vi "CallbackY.vi"(11 "IRQ Number":u8) -> ()   [LabVIEW 2017]
uses:
  <vilib>/myRIO/Instrument Drivers/Onboard IO/DIO/typedefs/DIO Reference.ctl
  <vilib>/myRIO/Common/Instrument Driver Framework/Utilities/typedefs/myRIO Generic Hardware Reference.ctl
  <vilib>/myRIO/Common/Instrument Driver Framework/Utilities/typedefs/Hardware Version Enum.ctl
  <vilib>/myRIO/Common/Instrument Driver Framework/Utilities/typedefs/myRIO v1.0 Reference.ctl
  <vilib>/myRIO/Common/Instrument Driver Framework/Utilities/typedefs/Generic FPGA Reference.ctl
  <vilib>/myRIO/Common/Instrument Driver Framework/myRIO v1.0/DIO/typedefs/DIO Channels List.ctl
  <vilib>/myRIO/Common/Instrument Driver Framework/myRIO v1.0/DIO/typedefs/DIO Channels Enum.ctl
  <vilib>/userdefined/High Color/nirio_resource_hc.ctl
  <vilib>/myRIO/Instrument Drivers/Onboard IO/DIO/vis/Write.vi
  <vilib>/myRIO/Common/Instrument Driver Framework/myRIO v1.0/DIO/vis/myRIO v1.1 Open DIO.vi
  <vilib>/myRIO/Common/Instrument Driver Framework/Utilities/vis/Is FPGA Ref Available.vi
  <vilib>/myRIO/Common/Instrument Driver Framework/Utilities/vis/Validate Channels.vi
  <vilib>/myRIO/Common/Instrument Driver Framework/myRIO v1.0/DIO/vis/myRIO v1.0 Reserve DIO.vi
  <vilib>/myRIO/Common/Instrument Driver Framework/myRIO v1.0/Resource Manager/vis/myRIO v1.0 Reserve Channel List.vi
  <vilib>/myRIO/Common/Instrument Driver Framework/myRIO v1.0/DIO/vis/myRIO v1.0 Build MUX Configuration DIO.vi
  <vilib>/myRIO/Common/Instrument Driver Framework/myRIO v1.0/Resource Manager/vis/myRIO v1.0 Reserve Channel.vi
  <vilib>/myRIO/Common/Instrument Driver Framework/myRIO v1.0/Resource Manager/vis/myRIO v1.0 Unreserve Channel.vi
  <vilib>/myRIO/Common/Instrument Driver Framework/myRIO v1.0/Resource Manager/vis/myRIO v1.0 Create Configuration List.vi
  <vilib>/myRIO/Common/Instrument Driver Framework/myRIO v1.0/Resource Manager/vis/myRIO v1.0 Build Mutex Name.vi
  <vilib>/myRIO/Common/Instrument Driver Framework/myRIO v1.0/DIO/vis/myRIO v1.0 Write DIO.vi
  <vilib>/Utility/error.llb/Error Cluster From Error Code.vi
  <vilib>/myRIO/Common/Instrument Driver Framework/myRIO v1.0/myRIO v1.0 Close.vi
  <vilib>/myRIO/Common/Instrument Driver Framework/myRIO v1.0/Resource Manager/vis/myRIO v1.0 Configure IO.vi
  <vilib>/myRIO/Common/Instrument Driver Framework/Utilities/vis/IO Manager.vi
  <vilib>/myRIO/Common/Instrument Driver Framework/Utilities/vis/Configuration Manager.vi
  <vilib>/myRIO/Common/Instrument Driver Framework/myRIO v1.0/myRIO v1.1 Open.vi
  <vilib>/Utility/VariantDataType/GetNumericInfo.vi
  Globales.vi
  <vilib>/myRIO/Instrument Drivers/Onboard IO/DIO/vis/myRIO DIO Open.xnode
  <vilib>/myRIO/Express VI/Onboard IO/DO/DO Express VI.xnode
  <vilib>/myRIO/Instrument Drivers/Onboard IO/DIO/DIO.lvlib
panel:
  out "Stop?":bool
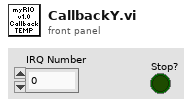
[diagram p1: front panel]
types:
  T1 = typedef "DIO.lvlib/DIO Reference.ctl" = cluster{"myRIO Reference":T2, "DIO Channels List":T6}
  T2 = typedef "myRIO Generic Hardware Reference.ctl" = cluster{"myRIO Model":T3, "myRIO Hardware Reference":T4}
  T3 = typedef "Hardware Version Enum.ctl" = enum16{"Unknown", "myRIO-1900", "myRIO-1950", "roboRIO", "NI ELVIS RIO CM"}
  T4 = typedef "myRIO v1.0 Reference.ctl" = cluster{"Generic FPGA Reference":T5, "Allow multiple opens":bool}
  T5 = typedef "Generic FPGA Reference.ctl" = refnum<k20>
  T6 = typedef "DIO Channels List.ctl" = T7[]
  T7 = typedef "DIO Channels Enum.ctl" = enum16{"Not Connected", "C/DIO0", "C/DIO1", "C/DIO2", "C/DIO3", "C/DIO4", "C/DIO5", "C/DIO6", "C/DIO7", "A/DIO0", "A/DIO1", "A/DIO2", "A/DIO3", "A/DIO4", "A/DIO5", "A/DIO6", "A/DIO7", "A/DIO8", "A/DIO9", "A/DIO10", "A/DIO11", "A/DIO12", "A/DIO13", "A/DIO14", "A/DIO15", "B/DIO0", "B/DIO1", "B/DIO2", "B/DIO3", "B/DIO4", "B/DIO5", "B/DIO6", "B/DIO7", "B/DIO8", "B/DIO9", "B/DIO10", "B/DIO11", "B/DIO12", "B/DIO13", "B/DIO14", "B/DIO15", "LED0", "LED1", "LED2", "LED3", "Button0", "DIO/DIO0", "DIO/DIO1", "DIO/DIO2", "DIO/DIO3", "DIO/DIO4", "DIO/DIO5", "DIO/DIO6", "DIO/DIO7", "DIO/DIO8", "DIO/DIO9", "SPI/CS0", "SPI/CS1", "SPI/CS2", "SPI/CS3", "LED RADIO (Green)", "LED RADIO (Red)", "LED COMM (Green)", "LED COMM (Red)", "LED MODE (Green)", "LED MODE (Red)"}
  T8 = typedef "nirio_resource_hc.ctl" = tag
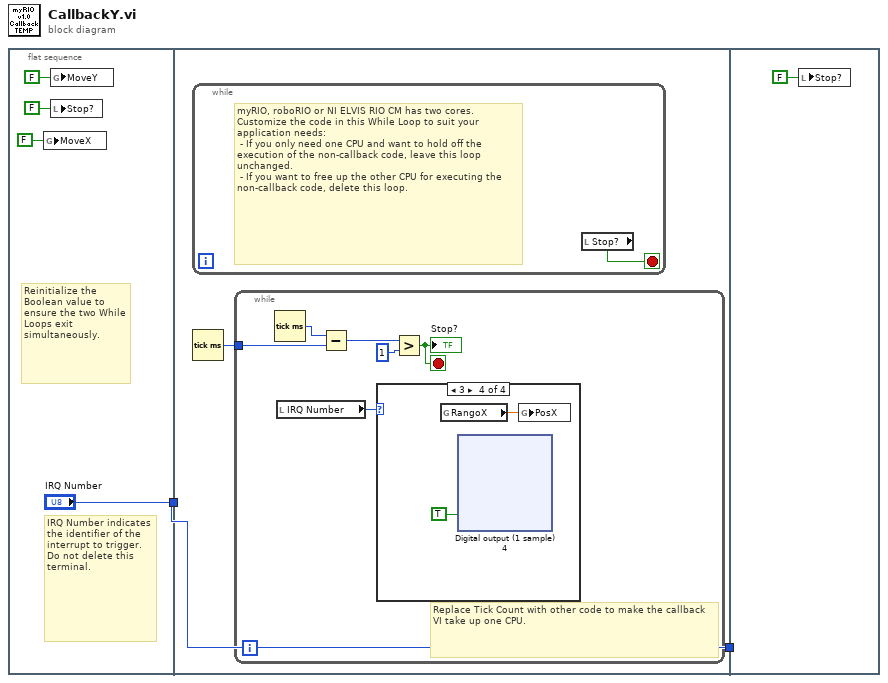
[diagram p0: block diagram]
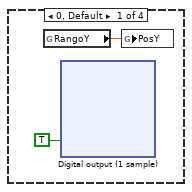
[diagram p2: hidden frame]
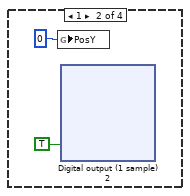
[diagram p3: hidden frame]
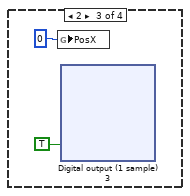
[diagram p4: hidden frame]
diagram:
  n1 = flat-sequence {
    tunnel: ["IRQ Number"] -> w2
    tunnel: [w8] -> w1
    tunnel: w2 -> [w8]
    tunnel: w1 -> [_]
    frame #0 {
      # "Reinitialize the Boolean value to ensure the two While Loops exit simultaneously."
      # "IRQ Number indicates the identifier of the interrupt to trigger. Do not delete this terminal."
      n2 = global write "Globales.vi" "MoveX"(FALSE) -> ()
      n3 = global write "Globales.vi" "MoveY"(FALSE) -> ()
      n4 = local write "Stop?"(FALSE ("Stop?")) -> ()
    }
    frame #1 {
      n5 = while {
        stop <- w9 stop-if-true
        # "myRIO, roboRIO or NI ELVIS RIO CM has two cores. Customize the code in this While Loop to suit your application needs:\n - If you only need one CPU and want to hold off the execution of the non-callback code, leave this loop unchanged.\n - If you want to free up the other CPU for executing the non-callback code, delete this loop."
        n6 = local read "Stop?"() -> (w9:bool)
      }
      n7 = Tick Count (ms)() -> (millisecond timer value=w7:u32)
      n8 = while {
        tunnel: w7 -> [w12]
        stop <- w11 stop-if-true
        # "Replace Tick Count with other code to make the callback VI take up one CPU."
        n9 = Tick Count (ms)() -> (millisecond timer value=w13:u32)
        n10 = local read "IRQ Number"() -> (w10:u8)
        n11 = Subtract(x=w13, y=w12) -> (x-y=w14:u32)
        n12 = case shown="3" w10 {
          frame 0, Default {
            n13 = global read "Globales.vi" "RangoY"() -> (w17:dbl)
            n14 = xnode "Digital output (1 sample)"("ON/OFF Y (A/DIO7 (Pin 25))"=TRUE) -> ()  [unwired: 1 in, 1 out]
            n15 = global write "Globales.vi" "PosY"(w17) -> ()
          }
          frame 1 {
            n16 = global write "Globales.vi" "PosY"(0) -> ()
            n17 = xnode "Digital output (1 sample) 2"("ON/OFF Y (A/DIO7 (Pin 25))"=TRUE) -> ()  [unwired: 1 in, 1 out]
          }
          frame 2 {
            n18 = global write "Globales.vi" "PosX"(0) -> ()
            n19 = xnode "Digital output (1 sample) 3"("ON/OFF Y (A/DIO4 (Pin 19))"=TRUE) -> ()  [unwired: 1 in, 1 out]
          }
          frame 3 {
            n20 = global read "Globales.vi" "RangoX"() -> (w128:dbl)
            n21 = xnode "Digital output (1 sample) 4"("ON/OFF X (A/DIO4 (Pin 19))"=TRUE) -> ()  [unwired: 1 in, 1 out]
            n22 = global write "Globales.vi" "PosX"(w128) -> ()
          }
        }
        n23 = Greater?(x=w14, y=u32 1) -> (0:w11:bool)
        "Stop?" <- w11
      }
    }
    frame #2 {
      n24 = local write "Stop?"(FALSE) -> ()
    }
  }
